vi "cg_Derivative Fletcher.vi"(2 "xi":dbl[](array[numeric]) format="%.2f", 3 "p":dbl[](array[numeric]) format="%.2f", 6 "ftol":dbl=0.0001 format="%.2e", 7 "function and data":T1, 8 "error in (no error)":errorcluster, 9 "c (start)":dbl=1.0 format="%.2f", 10 "b (start)":dbl=0.5 format="%.2f", 11 "a (start)":dbl format="%.2f") -> (0 "error out":errorcluster, 1 "x":dbl format="%.2f", 4 "minimum":dbl format="%.2f", 5 "number of function calls":i32)   [LabVIEW 2014, in "NI_Gmath.lvlib"]
uses:
  NI_Gmath.lvlib
  ucno_user function ref and data.ctl
  ucno_user objective function ref.ctl
  Unit Vector (DBL).vi
  Real Dot Product.vi
  NI_AALBase.lvlib
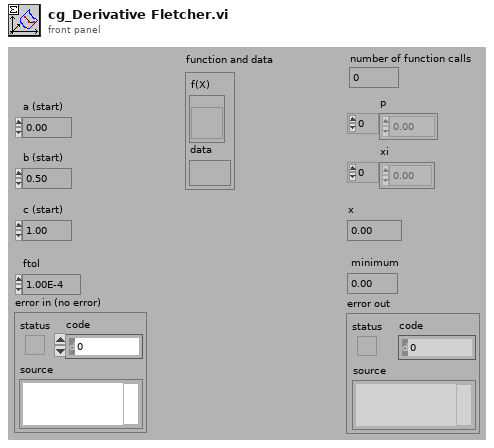
[diagram p1: front panel]
types:
  T1 = typedef "NI_Gmath.lvlib/ucno_user function ref and data.ctl" = cluster{"f(X)":T2, "data":variant}
  T2 = typedef "NI_Gmath.lvlib/ucno_user objective function ref.ctl" = refnum<vi>
  T3 = cluster{"objective function":bool, "gradient":bool}
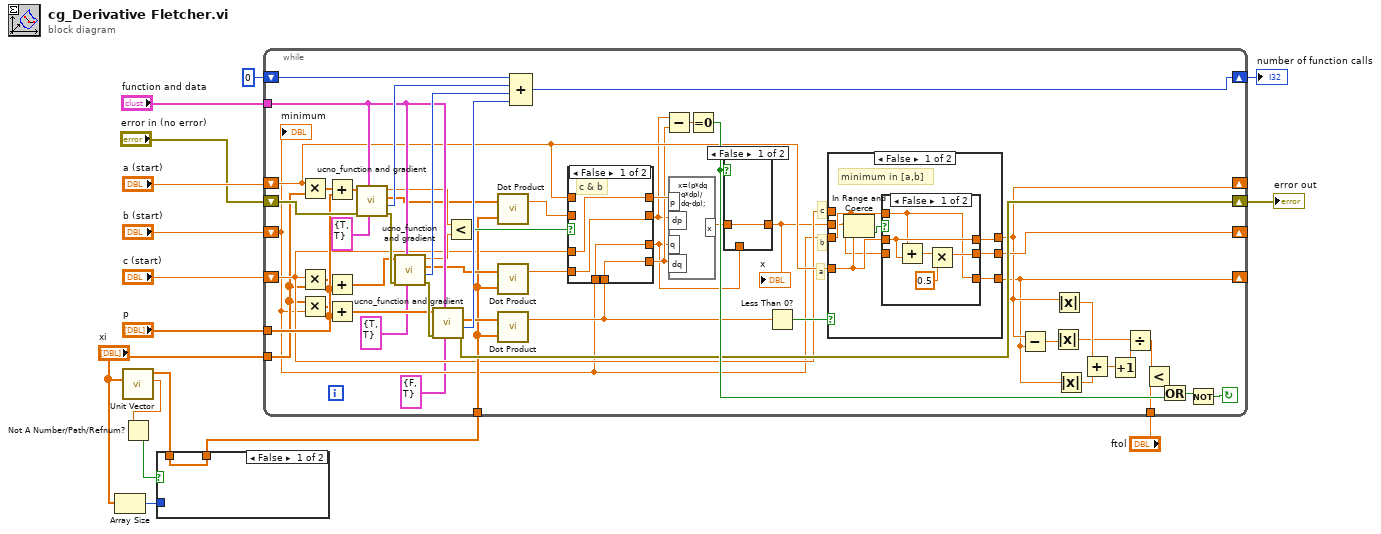
[diagram p0: block diagram]
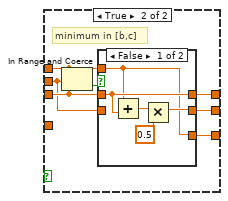
[diagram p5: hidden frame]
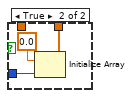
[diagram p7: hidden frame]
diagram:
  n1 = Array Size(array="xi") -> (size(s)=w7:i32)
  n2 = call-poly "Unit Vector.vi"("Input Vector"="xi") -> ("norm"=w10:dbl, "Unit Vector"=w9:dbl[])  [unwired: 8 in, 1 out]
  n3 = Not A Number/Path/Refnum?(number/path/refnum=w10) -> (NaN/Path/Refnum?=w11:bool)
  n4 = case shown="False" w11 {
    tunnel: w9 -> [w17 _]
    tunnel: [w17 w18] -> w6
    tunnel: w7 -> [_ w19]
    frame False {
    }
    frame True {
      n5 = Initialize Array(0.0, w19) -> (w18:dbl[])
    }
  }
  n6 = while {
    tunnel: w6 -> [w41]
    tunnel: "p" -> [w72]
    tunnel: "xi" -> [w38]
    tunnel: "ftol" -> [w54]
    shift-left: "c (start)" -> [w39]
    shift-right: [w61] -> _
    shift-left: "b (start)" -> [w36]
    shift-right: [w63] -> _
    shift-left: "a (start)" -> [w52]
    shift-right: [w62] -> _
    shift-right: [w70] -> w4
    shift-left: "error in (no error)" -> [w73]
    tunnel: "function and data" -> [w74]
    shift-right: [w21] -> w2
    shift-left: 0 -> [w22]
    stop <- w27 continue-if-true
    # "a"
    # "b"
    # "c"
    n7 = Multiply(x=w52, y=w38) -> (x*y=w51:dbl[])
    n8 = Multiply(x=w39, y=w38) -> (x*y=w40:dbl[])
    n9 = Multiply(x=w38, y=w36) -> (x*y=w47:dbl[])
    n10 = Add(x=w51, y=w72) -> (x+y=w50:dbl[])
    n11 = Add(x=w40, y=w72) -> (x+y=w37:dbl[])
    n12 = Add(x=w47, y=w72) -> (x+y=w45:dbl[])
    n13 = call "ucno_function and gradient.vi"("output control"=T3 {"objective function"=TRUE, "gradient"=TRUE}, "function and data"=w74, "error in (no error)"=w73, "X"=w50) -> ("error out"=w69:errorcluster, "number of function calls"=w77:i32, "gradient"=w49:dbl[], "f(X)"=w67:dbl)  [unwired: 4 in]
    n14 = call "ucno_function and gradient.vi"("output control"=T3 {"objective function"=TRUE, "gradient"=TRUE}, "function and data"=w74, "error in (no error)"=w69, "X"=w37) -> ("error out"=w68:errorcluster, "number of function calls"=w75:i32, "gradient"=w42:dbl[], "f(X)"=w66:dbl)  [unwired: 4 in]
    n15 = call "ucno_function and gradient.vi"("output control"=T3 {"objective function"=FALSE, "gradient"=TRUE}, "function and data"=w74, "error in (no error)"=w68, "X"=w45) -> ("error out"=w70:errorcluster, "number of function calls"=w76:i32, "gradient"=w46:dbl[])  [unwired: 4 in, 1 out]
    n16 = Less?(x=w67, y=w66) -> (x < y?=w65:bool)
    n17 = call-poly "Dot Product.vi"("Y Vector"=w41, "X Vector"=w49) -> ("X * Y"=w48:dbl)  [unwired: 1 out]
    n18 = call-poly "Dot Product.vi"("Y Vector"=w41, "X Vector"=w42) -> ("X * Y"=w43:dbl)  [unwired: 1 out]
    n19 = call-poly "Dot Product.vi"("Y Vector"=w41, "X Vector"=w46) -> ("X * Y"=w44:dbl)  [unwired: 1 out]
    n20 = Compound Arithmetic op=ADD(w22, w77, w75, w76) -> (w21:i32)
    n21 = case shown="False" w65 {
      tunnel: w39 -> [w81 _]
      tunnel: w44 -> [w82 w84]
      tunnel: w43 -> [w80 _]
      tunnel: w48 -> [_ w86]
      tunnel: w52 -> [_ w87]
      tunnel: [w81 w87] -> w35
      tunnel: [w80 w86] -> w33
      tunnel: w36 -> [w83 w85]
      tunnel: [w83 w85] -> w29
      tunnel: [w82 w84] -> w34
      frame False {
        # "c & b"
      }
      frame True {
        # "a & b"
      }
    }
    n22 = Subtract(x=w33, y=w34) -> (x-y=w32:dbl)
    n23 = formula code="x=(p*dq-q*dp)/(dq-dp);"("p"=w35, "q"=w29, "dp"=w33, "dq"=w34) -> ("x"=w31:dbl)
    n24 = Equal To 0?(x=w32) -> (x = 0?=w71:bool)
    n25 = case shown="False" w71 {
      tunnel: w31 -> [w78 _]
      tunnel: [w78 w79] -> w30
      tunnel: w29 -> [_ w79]
      frame False {
      }
      frame True {
      }
    }
    "x" <- w30
    n26 = Less Than 0?(x=w44) -> (x < 0?=w64:bool)
    n27 = case shown="False" w64 {
      tunnel: w30 -> [w90 w106]
      tunnel: w36 -> [w93 w108]
      tunnel: w39 -> [_ w104]
      tunnel: w52 -> [w91 _]
      tunnel: [w92 w107] -> w62
      tunnel: [w89 w105] -> w63
      tunnel: [w88 w103] -> w61
      frame False {
        # "minimum in [a,b]"
        n28 = In Range and Coerce(upper limit=w93, x=w90, lower limit=w91) -> (In Range?=w94:bool)  [unwired: 1 out]
        n29 = case shown="False" w94 {
          tunnel: w91 -> [w97 w102]
          tunnel: [w97 w102] -> w92
          tunnel: w90 -> [_ w101]
          tunnel: [w96 w101] -> w89
          tunnel: w93 -> [w95 w100]
          tunnel: [w95 w100] -> w88
          frame False {
            n30 = Add(x=w95, y=w97) -> (x+y=w99:dbl)
            n31 = Multiply(x=w99, y=0.5) -> (x*y=w96:dbl)
          }
          frame True {
          }
        }
      }
      frame True {
        # "minimum in [b,c]"
        n32 = In Range and Coerce(upper limit=w104, x=w106, lower limit=w108) -> (In Range?=w109:bool)  [unwired: 1 out]
        n33 = case shown="False" w109 {
          tunnel: w108 -> [w112 w117]
          tunnel: [w112 w117] -> w107
          tunnel: w106 -> [_ w116]
          tunnel: [w111 w116] -> w105
          tunnel: w104 -> [w110 w115]
          tunnel: [w110 w115] -> w103
          frame False {
            n34 = Add(x=w110, y=w112) -> (x+y=w114:dbl)
            n35 = Multiply(x=w114, y=0.5) -> (x*y=w111:dbl)
          }
          frame True {
          }
        }
      }
    }
    n36 = Subtract(x=w62, y=w61) -> (x-y=w53:dbl)
    n37 = Absolute Value(x=w53) -> (abs(x)=w56:dbl)
    n38 = Absolute Value(x=w62) -> (abs(x)=w60:dbl)
    n39 = Absolute Value(x=w61) -> (abs(x)=w59:dbl)
    n40 = Add(x=w60, y=w59) -> (x+y=w58:dbl)
    n41 = Increment(x=w58) -> (x+1=w57:dbl)
    n42 = Divide(x=w56, y=w57) -> (x/y=w55:dbl)
    n43 = Less?(x=w55, y=w54) -> (x < y?=w28:bool)
    n44 = Or(x=w28, y=w71) -> (x .or. y?=w26:bool)
    n45 = Not(x=w26) -> (.not. x?=w27:bool)
    "minimum" <- w36
  }
  "error out" <- w4
  "number of function calls" <- w2
